vi "XY2JointAngles.vi"(9 "y":dbl, 10 "x":dbl) -> (1 "Corrected joint 2":dbl, 2 "Corrected joint 1":dbl)   [LabVIEW 2023]
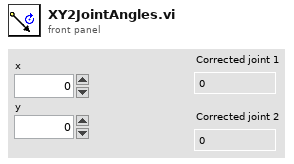
[diagram p1: front panel]
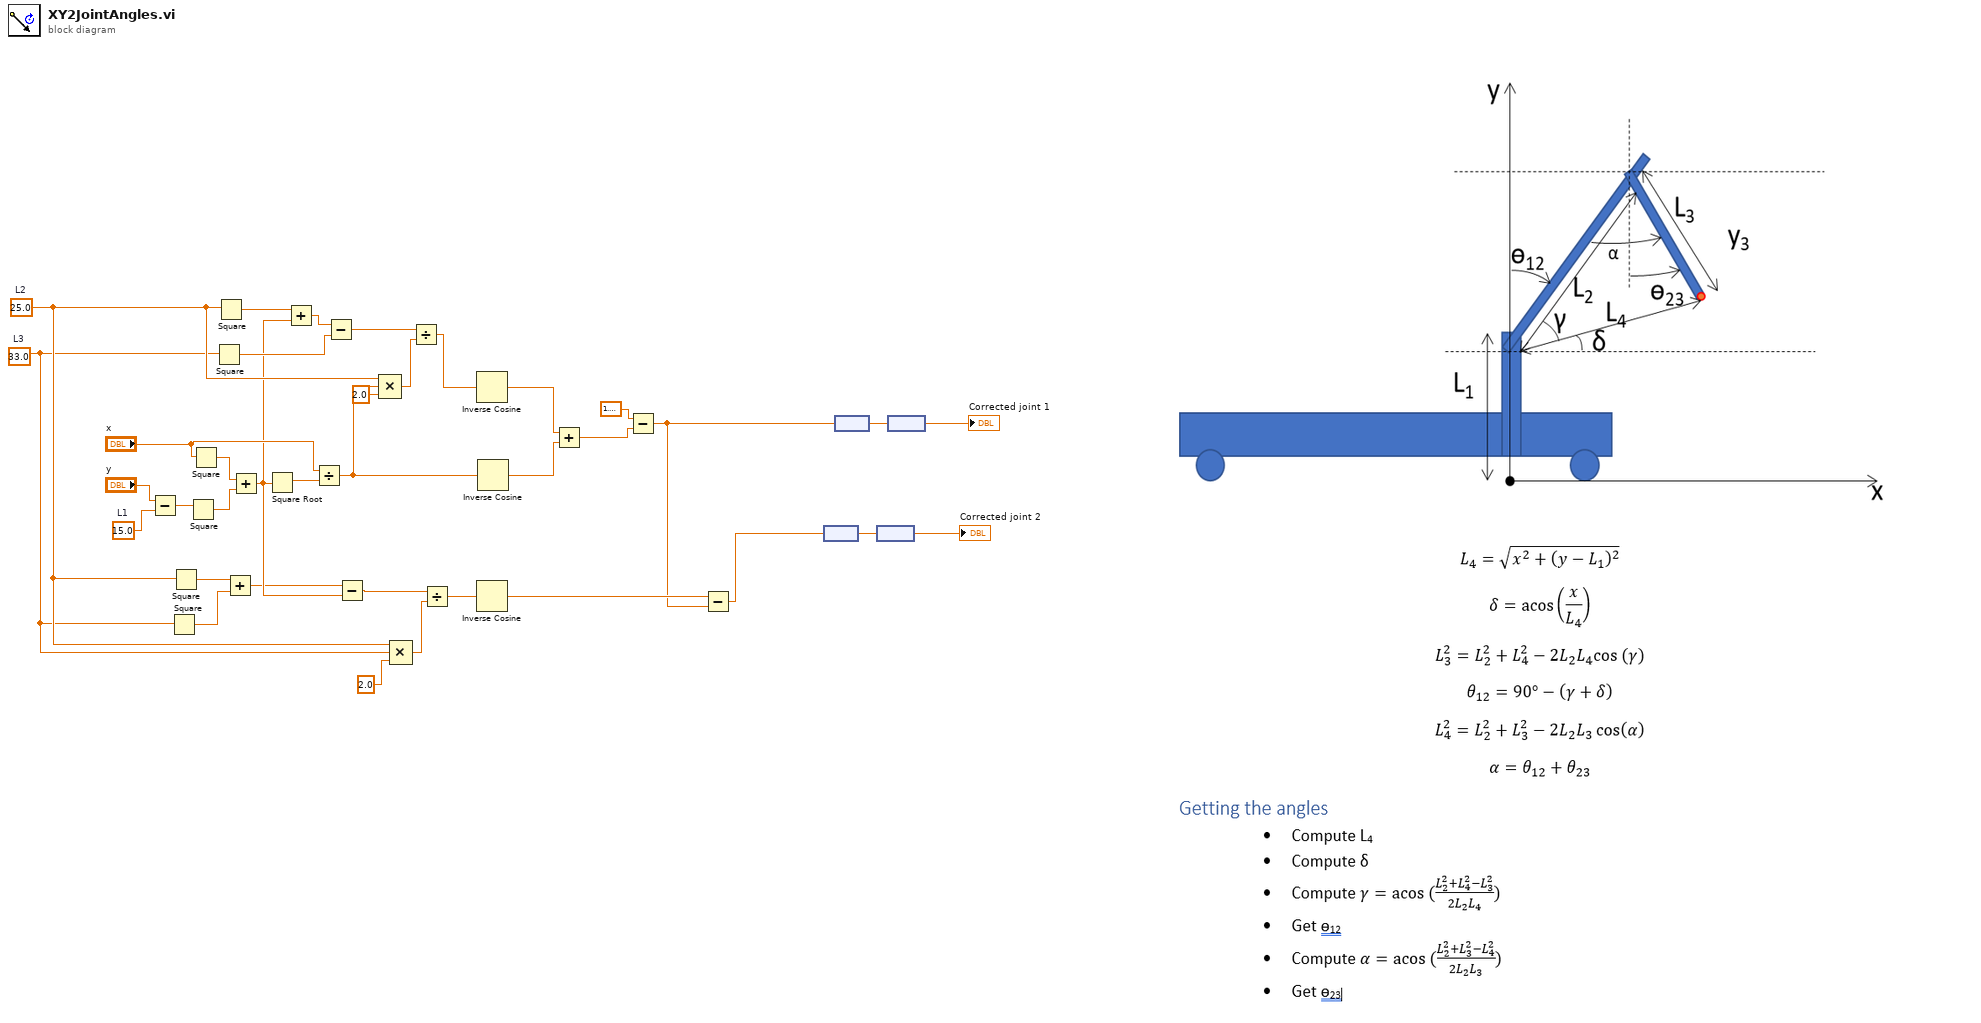
[diagram p0: block diagram]
diagram:
  w5 = 25.0  # L2
  w4 = 33.0  # L3
  w31 = 15.0  # L1
  n1 = Subtract(x="y", y=w31) -> (x-y=w30:dbl)
  n2 = Square(x=w4) -> (x^2=w3:dbl)
  n3 = Square(x=w5) -> (x^2=w6:dbl)
  n4 = Square(x=w30) -> (x^2=w28:dbl)
  n5 = Square(x="x") -> (x^2=w29:dbl)
  n6 = Square(x=w4) -> (x^2=w19:dbl)
  n7 = Square(x=w5) -> (x^2=w21:dbl)
  n8 = Add(x=w6, y=w3) -> (x+y=w1:dbl)
  n9 = Add(x=w29, y=w28) -> (x+y=w2:dbl)
  n10 = Square Root(x=w2) -> (sqrt(x)=w27:dbl)
  n11 = Add(x=w21, y=w2) -> (x+y=w20:dbl)
  n12 = Divide(x="x", y=w27) -> (x/y=w16:dbl)
  n13 = Subtract(x=w20, y=w19) -> (x-y=w18:dbl)
  n14 = Subtract(x=w1, y=w2) -> (x-y=w8:dbl)
  n15 = Compound Arithmetic op=MULTIPLY(w5, w16, 2.0 ("value")) -> (w14:dbl)
  n16 = Compound Arithmetic op=MULTIPLY(w5, w4, 2.0 ("value")) -> (w10:dbl)
  n17 = Divide(x=w18, y=w14) -> (x/y=w17:dbl)
  n18 = Divide(x=w8, y=w10) -> (x/y=w7:dbl)
  n19 = Inverse Cosine(1:w17) -> (0:w24:dbl)
  n20 = Inverse Cosine(1:w7) -> (0:w13:dbl)
  n21 = Inverse Cosine(1:w16) -> (0:w25:dbl)
  n22 = Add(x=w24, y=w25) -> (x+y=w22:dbl)
  n23 = Subtract(x=1.5707963267948966, y=w22) -> (x-y=w12:dbl)
  n24 = Subtract(x=w13, y=w12) -> (x-y=w11:dbl)
  n25 = node(w11) -> (w35:dbl[unit])
  n26 = node(w12) -> (w36:dbl[unit])
  n27 = node(w35) -> (→"Corrected joint 2":dbl)
  n28 = node(w36) -> (→"Corrected joint 1":dbl)
